vi "CopyROIPitch.vi"(6 "Root":path, 8 "error in (no error)":errorcluster, 9 "ROI List":i32[](array[numeric]), 10 "ROIs":T1[](array[typedef]) {"Contours"."Type" items=["No Selection", "Point", "Line", "Rectangle", "Oval", "Polygon", "Freehand Region", "Annulus", "Unused2", "Unused3", "Broken Line", "Freehand Line", "Rotated Rectangle"]}) -> (0 "error out":errorcluster)   [LabVIEW 2019]
uses:
  Controls/ROI_List_Action.ctl
  Analysis/Controls/Parttern Match/Analysis_PatternMatch_Parameter.ctl
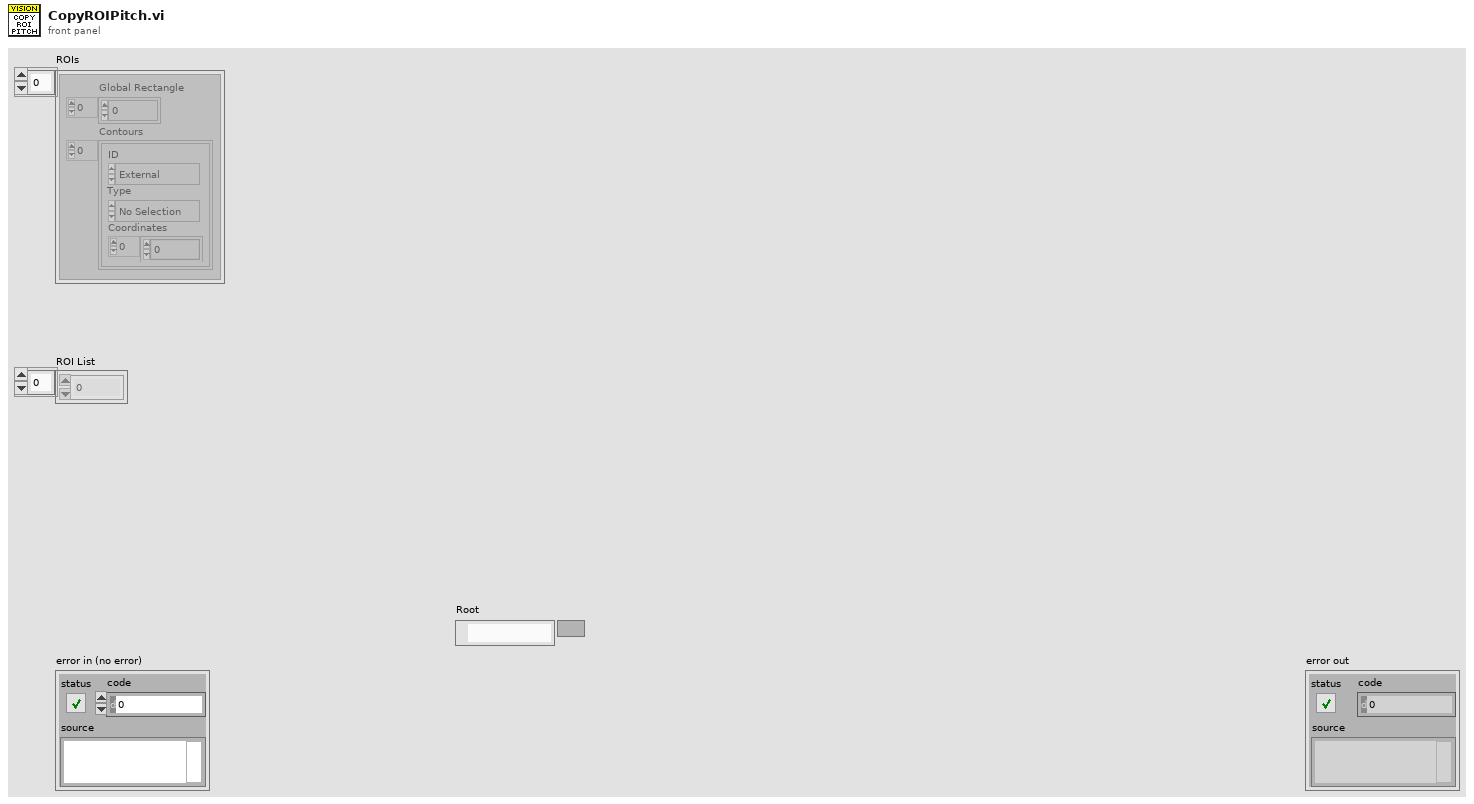
[diagram p1: front panel]
types:
  T1 = typedef "ROI Descriptor" = cluster{"Global Rectangle":i32[], "Contours":cluster{"ID":enum32{"External", "Internal"}, "Type":u32, "Coordinates":i32[]}[]}
  T2 = typedef "ROI_List_Action.ctl" = enum16{"Init", "Add ROI", "Delete ROI", "Get All ROI", "Get Specific ROI", "Set Analysis Setting", "Set Process Setting", "Replace All Entries", "ROIEntryBackup", "ROIEntryBackupClear", "ROIEntryReturn"}
  T3 = typedef "Vision_DataEntry.ctl" = cluster{"vROIName":string, "vROIContour":cluster{"Contour Type":u32, "ROI Type":u32, "Points":i32[]}, "ProcessSetting":T4[], "Analysis_Setting":T6}
  T4 = typedef "Process_Setting.ctl" = cluster{"Enum_PreProcess":T5, "Parameter":string}
  T5 = typedef "VisionProcessName.ctl" = enum16{"*CamParameter*", "CamAttributes", "*Preprocess*", "CG_Brightness", "C_Plane Extraction", "C_Threshold", "G_Lookup Table", "G_Threshold"}
  T6 = typedef "Analysis_Setting.ctl" = cluster{"PreProcess":T7, "Parameter":string}
  T7 = typedef "VisionProcessName.ctl" = enum16{"*CamParameter*", "CamAttributes", "*Preprocess*", "CG_Brightness", "C_Plane Extraction", "C_Threshold", "G_Lookup Table", "G_Threshold", "B_Image Inversion", "*Algorithm*", "CG_Histogram", "C_Color Matching", "C_Color Pattern Matching", "G_PatternMatch", "CG_Find Straight Edge", "CG_Adv. Find Straight Edge", "CG_Find Circular Edge", "G_Max Clamp", "G_Clamp (Rake)", "G_Pattern Matching"}
  T8 = cluster{"Contour Type":u32, "ROI Type":u32, "Points":i32[]}
  T9 = typedef "Analysis_PatternMatch_Parameter.ctl" = cluster{"Algorithm":i32, "Match Parameters":cluster{"Number of Matches Requested":i32, "Minimum Match Score":sgl, "Angle Ranges":cluster{"Start Angle":sgl, "End Angle":sgl}[]}, "ROI Descriptor":T1, "Advanced Options":cluster{"Item":u16, "Value":dbl}[], "Template path":string, "XOffset":i32, "YOffset":i32}
  T10 = cluster{"ID":enum32{"External", "Internal"}, "Type":u32, "Coordinates":i32[]}[]
  T11 = cluster{"ID":enum32{"External", "Internal"}, "Type":u32, "Coordinates":i32[]}
  T12 = typedef "Vision_DataEntry.ctl" = cluster{"vROIName":string, "vROIContour":cluster{"Contour Type":u32, "ROI Type":u32, "Points":i32[]}, "ProcessSetting":T4[], "Analysis_Setting":T13}
  T13 = typedef "Analysis_Setting.ctl" = cluster{"PreProcess":T14, "Parameter":string}
  T14 = typedef "V_Analysis_Type.ctl" = enum16{"None", "C_Color Pattern Matching", "G_PatternMatching", "G_ShapeDectect", "G_GeometricMatch", "B_Area Check"}
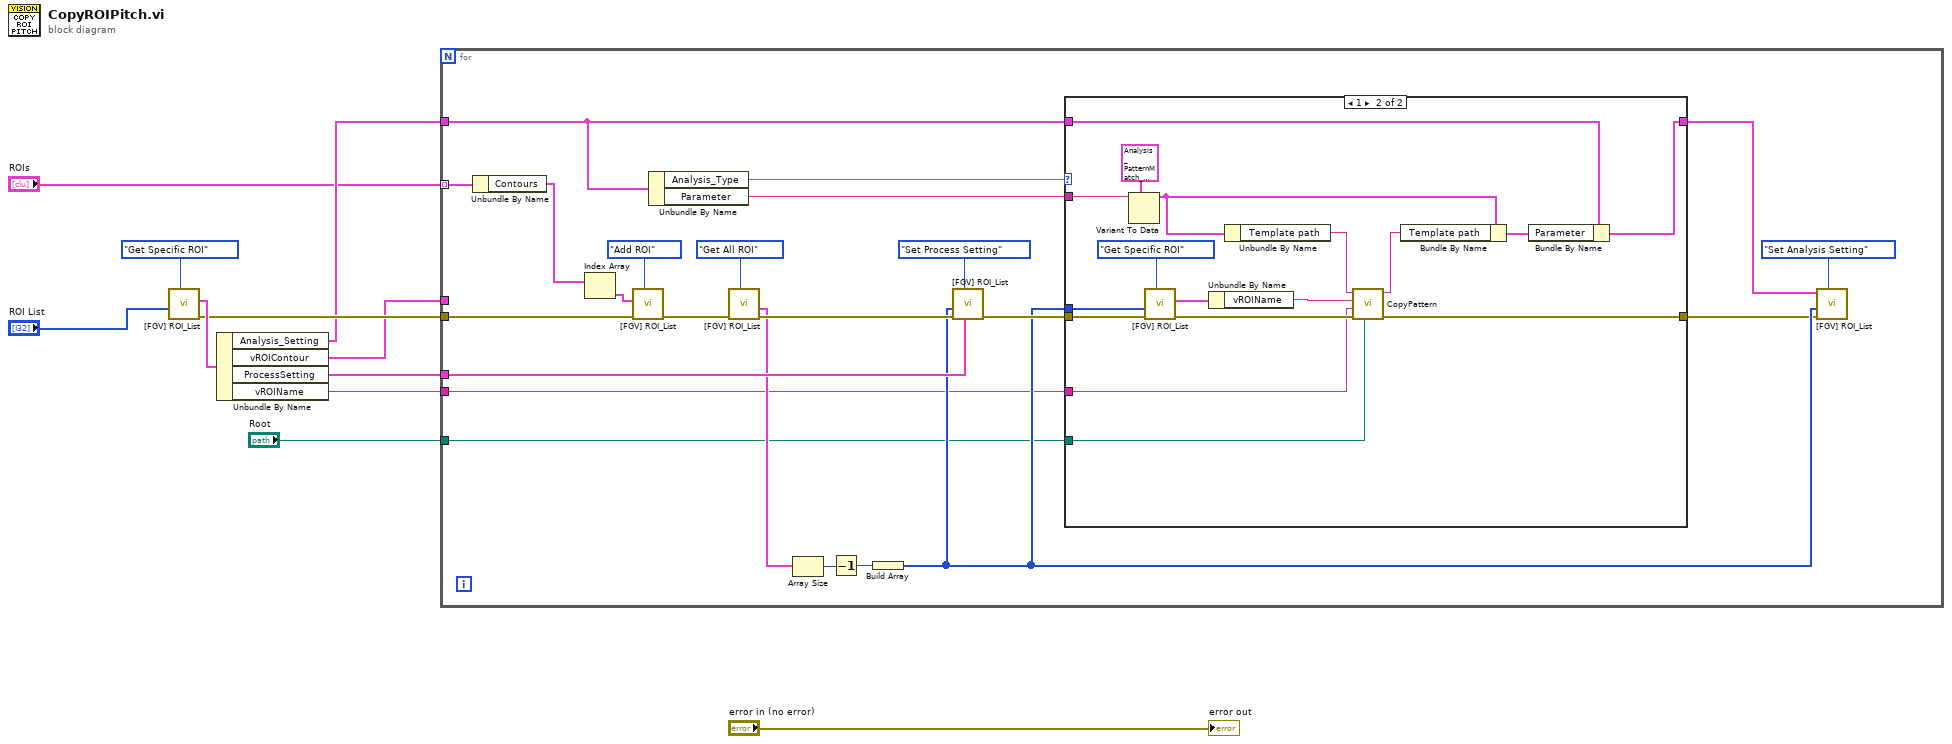
[diagram p0: block diagram]
diagram:
  n1 = call "[FGV] ROI_List.vi"("Action"=ROI_List_Action."Get Specific ROI", "ROIs_Index"="ROI List") -> ("error out"=w8:errorcluster, "ROI Entry"=w10:T3)  [unwired: 7 in, 1 out]
  n2 = Unbundle By Name(w10) -> ("Analysis_Setting"=w6:T6, "vROIContour"=w7:T8, "ProcessSetting"=w5:T4[], "vROIName"=w4:string)
  n3 = for {
    tunnel: w5 -> [w32]
    tunnel: w8 -> [w30]
    tunnel: w7 -> [_]
    tunnel: w6 -> [w18]
    tunnel: w4 -> [w16]
    tunnel: "Root" -> [w15]
    tunnel: "ROIs" -> [w14] mode=indexing
    n4 = Unbundle By Name(w14) -> ("Contours"=w13:T10)
    n5 = Index Array(array=w13) -> (element=w12:T11)  [unwired: 1 in]
    n6 = call "[FGV] ROI_List.vi"("Action"=ROI_List_Action."Add ROI", "error in (no error)"=w30, "ROI_To_Add"=w12) -> ("error out"=w28:errorcluster)  [unwired: 6 in, 2 out]
    n7 = Unbundle By Name(w18) -> ("Analysis_Type"=w22, "Parameter"=w24:string)
    n8 = call "[FGV] ROI_List.vi"("Action"=ROI_List_Action."Get All ROI", "error in (no error)"=w28) -> ("error out"=w27:errorcluster, "All ROI"=w26:T12[])  [unwired: 7 in, 1 out]
    n9 = Array Size(array=w26) -> (size(s)=w25:i32)
    n10 = Decrement(x=w25) -> (x-1=w23:i32)
    n11 = Build Array(w23) -> (w20:i32[])
    n12 = call "[FGV] ROI_List.vi"("ProcessSetting"=w32, "Action"=ROI_List_Action."Set Process Setting", "error in (no error)"=w27, "ROIs_Index"=w20) -> ("error out"=w21:errorcluster)  [unwired: 5 in, 2 out]
    n13 = case shown="1" w22 {
      tunnel: w24 -> [_ w52]
      tunnel: w21 -> [w35 w49]
      tunnel: w20 -> [_ w48]
      tunnel: [w35 w37] -> w19
      tunnel: w18 -> [w36 w46]
      tunnel: [w36 w44] -> w17
      tunnel: w16 -> [_ w39]
      tunnel: w15 -> [_ w38]
      frame Default {
      }
      frame 1 {
        n14 = Variant To Data(type=T9 {"Algorithm"=2, "Match Parameters"={"Number of Matches Requested"=1, "Minimum Match Score"=750.0, "Angle Ranges"=[]}, "ROI Descriptor"={"Global Rectangle"=[], "Contours"=[]}, "Advanced Options"=[{"Item"=1, "Value"=1.0}, {"Item"=103, "Value"=1.0}], "Template path"="", "XOffset"=0, "YOffset"=0} ("PatternMatchParameter"), Variant=w52) -> (data=w51:T9)  [unwired: 1 in, 1 out]
        n15 = call "[FGV] ROI_List.vi"("Action"=ROI_List_Action."Get Specific ROI", "error in (no error)"=w49, "ROIs_Index"=w48) -> ("error out"=w43:errorcluster, "ROI Entry"=w47:T3)  [unwired: 6 in, 1 out]
        n16 = Unbundle By Name(w47) -> ("vROIName"=w40:string)
        n17 = Unbundle By Name(w51) -> ("Template path"=w42:string)
        n18 = call "CopyPattern.vi"("Root"=w38, "error in (no error)"=w43, "SourceName"=w39, "CopyName"=w40, "SourcePatternPath"=w42) -> ("error out"=w37:errorcluster, "CopyPatternPath"=w41:string)  [unwired: 5 in]
        n19 = Bundle By Name(cluster=w51, "Template path"=w41) -> (w45:T9)
        n20 = Bundle By Name(cluster=w46, "Parameter"=w45) -> (w44:T6)
      }
    }
    n21 = call "[FGV] ROI_List.vi"("Action"=ROI_List_Action."Set Analysis Setting", "error in (no error)"=w19, "ROIs_Index"=w20, "Analysis_Setting"=w17) -> ()  [unwired: 5 in, 3 out]
  }
  "error out" <- "error in (no error)"
